vi "Build Calibration Marker Board Points.vi"(1 "Marker Size":cluster{"Width":i32, "Height":i32}, 2 "Top Left Point":T1) -> (0 "Marker Corners - AprilTag Detector Order":T1[](array[typedef]))   [LabVIEW 2020, in "AR Example.lvlib" / "App.lvclass"]
uses:
  App.lvclass
  g_ar_toolkit.common/Object Point (Float).ctl
  App.lvclass/App.ctl
  g_ar_toolkit.common/g_ar_toolkit.common.lvlib
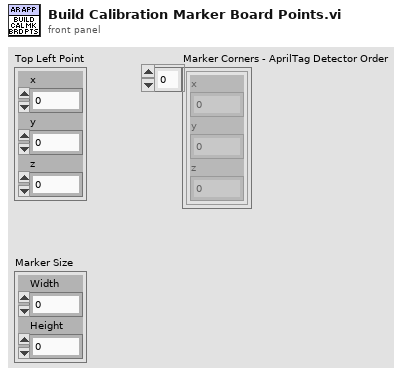
[diagram p1: front panel]
types:
  T1 = typedef "g_ar_toolkit.common.lvlib/Object Point (Float).ctl" = cluster{"x":dbl, "y":dbl, "z":dbl}
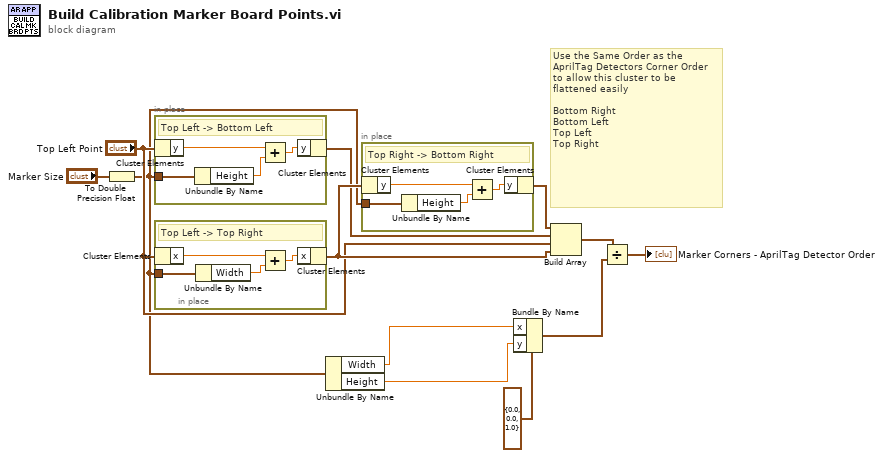
[diagram p0: block diagram]
diagram:
  # "Use the Same Order as the AprilTag Detectors Corner Order to allow this cluster to be flattened easily\n\nBottom Right\nBottom Left\nTop Left\nTop Right"
  n1 = To Double Precision Float(number="Marker Size") -> (double precision float=w4:cluster{"Width":dbl, "Height":dbl})
  n2 = in-place {
    in-place-border: w4 -> [w16]
    # "Top Left -> Bottom Left"
    n3 = in-place-cluster #1("Top Left Point") -> ("y"=w14:dbl)
    n4 = Unbundle By Name(w16) -> ("Height"=w15:dbl)
    n5 = Add(x=w14, y=w15) -> (x+y=w13:dbl)
    n6 = in-place-cluster #1("y"=w13) -> (w7:T1)
  }
  n7 = in-place {
    in-place-border: w4 -> [w20]
    # "Top Left -> Top Right"
    n8 = in-place-cluster #2("Top Left Point") -> ("x"=w18:dbl)
    n9 = Unbundle By Name(w20) -> ("Width"=w19:dbl)
    n10 = Add(x=w18, y=w19) -> (x+y=w17:dbl)
    n11 = in-place-cluster #2("x"=w17) -> (w10:T1)
  }
  n12 = Unbundle By Name(w4) -> ("Width"=w3:dbl, "Height"=w2:dbl)
  n13 = in-place {
    in-place-border: w4 -> [w24]
    # "Top Right -> Bottom Right"
    n14 = in-place-cluster #3(w10) -> ("y"=w22:dbl)
    n15 = Unbundle By Name(w24) -> ("Height"=w23:dbl)
    n16 = Add(x=w22, y=w23) -> (x+y=w21:dbl)
    n17 = in-place-cluster #3("y"=w21) -> (w9:T1)
  }
  n18 = Bundle By Name(cluster=T1 {"x"=0.0, "y"=0.0, "z"=1.0}, "x"=w3, "y"=w2) -> (w1:T1)
  n19 = Build Array(w9, w7, "Top Left Point", w10) -> (w11:T1[])
  n20 = Divide(x=w11, y=w1) -> (x/y=→"Marker Corners - AprilTag Detector Order":T1[])
